vi "Golden Section 1D_core(VI).vi"(4 "sign":i32(ring) items=["y=f(x)", "y=-f(x)"], 5 "accuracy":dbl=1e-08 format="%.0e", 6 "data":variant, 7 "f(x)":T1, 8 "error in":i32, 9 "c (start)":dbl format="%.2f", 10 "b (start)":dbl format="%.2f", 11 "a (start)":dbl format="%.2f") -> (0 "error out":i32, 1 "ticks":u32, 2 "f(minimum)":dbl format="%.2f", 3 "minimum":dbl format="%.2f")   [LabVIEW 2014, in "NI_Gmath.lvlib"]
uses:
  NI_Gmath.lvlib
  functionRefnum.ctl
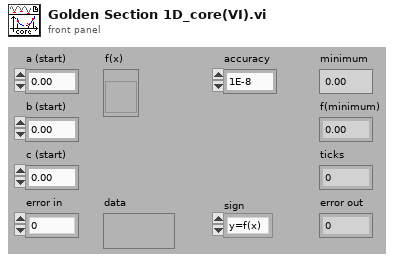
[diagram p1: front panel]
types:
  T1 = typedef "NI_Gmath.lvlib/functionRefnum.ctl" = refnum<vi>
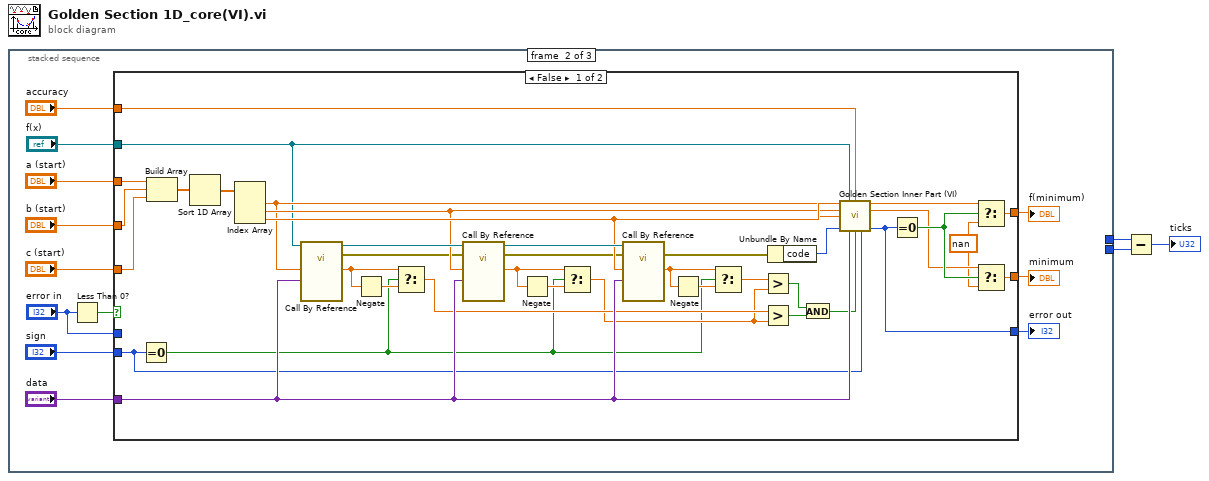
[diagram p0: block diagram]
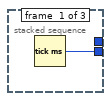
[diagram p2: hidden frame]
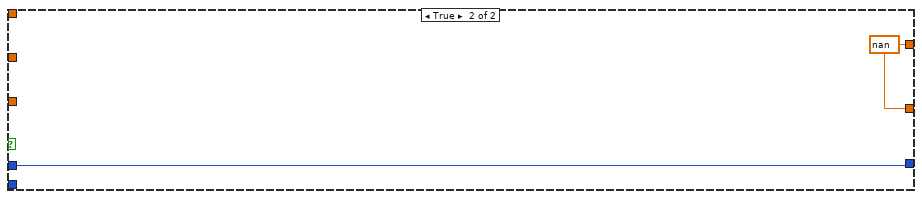
[diagram p3: hidden frame]
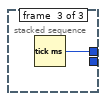
[diagram p4: hidden frame]
diagram:
  n1 = stacked-sequence {
    tunnel: [w4 _ _] -> w2
    tunnel: [_ _ w57] -> w1
    frame #0 {
      n2 = Tick Count (ms)() -> (millisecond timer value=w4:u32)
    }
    frame #1 {
      n3 = Less Than 0?(x="error in") -> (x < 0?=w13:bool)
      n4 = case shown="False" w13 {
        tunnel: [w52 w55] -> w16
        tunnel: [w48 w56] -> w15
        tunnel: [w45 w56] -> w14
        tunnel: "error in" -> [_ w55]
        tunnel: "f(x)" -> [w35 _]
        tunnel: "accuracy" -> [w31 _]
        tunnel: "a (start)" -> [w30 _]
        tunnel: "b (start)" -> [w29 _]
        tunnel: "c (start)" -> [w28 _]
        tunnel: "data" -> [w54 _]
        tunnel: "sign" -> [w17 _]
        frame False {
          w44 = nan
          n5 = Equal To 0?(x=w17) -> (x = 0?=w18:bool)
          n6 = Build Array(w30, w29, w28) -> (w51:dbl[])
          n7 = Sort 1D Array(array=w51) -> (sorted array=w41:dbl[])
          n8 = Index Array(array=w41) -> (element #1=w38:dbl, element #2=w39:dbl, element #3=w40:dbl)  [unwired: 3 in]
          n9 = call-by-ref "?"(reference=w35, "Variant"=w54, "x"=w38) -> (reference out=w42:T1, error out=w33:errorcluster, 2:"f(x)"=w26:dbl)  [unwired: 4 in]
          n10 = Negate(x=w26) -> (-x=w27:dbl)
          n11 = Select(t=w26, s=w18, f=w27) -> (s? t:f=w25:dbl)
          n12 = call-by-ref "?"(reference=w42, error in=w33, "Variant"=w54, "x"=w39) -> (reference out=w43:T1, error out=w34:errorcluster, 2:"f(x)"=w22:dbl)  [unwired: 3 in]
          n13 = Negate(x=w22) -> (-x=w24:dbl)
          n14 = Select(t=w22, s=w18, f=w24) -> (s? t:f=w23:dbl)
          n15 = call-by-ref "?"(reference=w43, error in=w34, "Variant"=w54, "x"=w40) -> (error out=w32:errorcluster, "f(x)"=w19:dbl)  [unwired: 3 in, 1 out]
          n16 = Negate(x=w19) -> (-x=w21:dbl)
          n17 = Select(t=w19, s=w18, f=w21) -> (s? t:f=w20:dbl)
          n18 = Greater?(x=w20, y=w23) -> (0:w53:bool)
          n19 = Greater?(x=w25, y=w23) -> (0:w50:bool)
          n20 = Unbundle By Name(w32) -> ("code"=w36:i32)
          n21 = And(x=w53, y=w50) -> (x .and. y?=w37:bool)
          n22 = call "Golden Section Inner Part (VI).vi"("a (start)"=w40, "f(x)"=w35, "accuracy"=w31, "b (start)"=w39, "c (start)"=w38, "error in"=w36, "data"=w54, "case"=w37, "sign"=w17) -> ("minimum"=w49:dbl, "f(minimum)"=w46:dbl, "error out"=w52:i32)  [unwired: 4 out]
          n23 = Equal To 0?(x=w52) -> (x = 0?=w47:bool)
          n24 = Select(t=w49, s=w47, f=w44) -> (s? t:f=w48:dbl)
          n25 = Select(t=w46, s=w47, f=w44) -> (s? t:f=w45:dbl)
        }
        frame True {
          w56 = nan ("minimum")
        }
      }
      "f(minimum)" <- w15
      "minimum" <- w14
      "error out" <- w16
    }
    frame #2 {
      n26 = Tick Count (ms)() -> (millisecond timer value=w57:u32)
    }
  }
  n27 = Subtract(x=w1, y=w2) -> (x-y=→"ticks":u32)
